vi "Read Append Numeric.vi"(11 "StringIncrement":refnum<class "StringIncrement.Alphabetical.lvclass">) -> (2 "Append Numeric":u32, 3 "StringIncrement out":refnum<class "StringIncrement.Alphabetical.lvclass">)   [LabVIEW 2014]
uses:
  StringIncrement.Alphabetical.lvclass
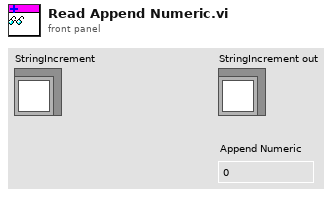
[diagram p1: front panel]
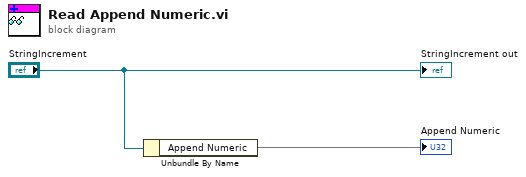
[diagram p0: block diagram]
diagram:
  n1 = Unbundle By Name("StringIncrement") -> ("Append Numeric"=→"Append Numeric")
  "StringIncrement out" <- "StringIncrement"
